vi "Prober_LoadUnload.vi"(8 "error in (no error)":errorcluster, 11 "TeslaVeloxProbeStation in":refnum<class "TeslaVeloxProbeStation.lvclass">) -> (0 "error out":errorcluster, 2 "Home or Load?":enum16{"Measure", "Load"}(ring), 3 "TeslaVeloxProbeStation out":refnum<class "TeslaVeloxProbeStation.lvclass">)   [LabVIEW 2018, in "TeslaVeloxProbeStation.lvclass"]
uses:
  TeslaVeloxProbeStation.lvclass
  Desktop/Kvasnicka/test_labview_library/Integration_toolkit_library/CascadeProbestation.lvlib
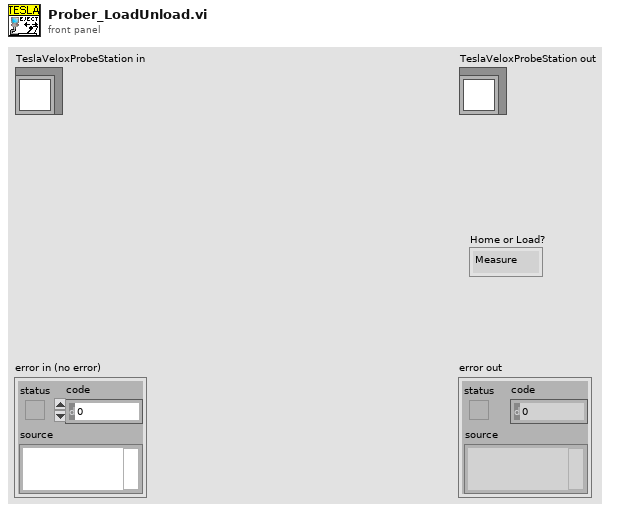
[diagram p1: front panel]
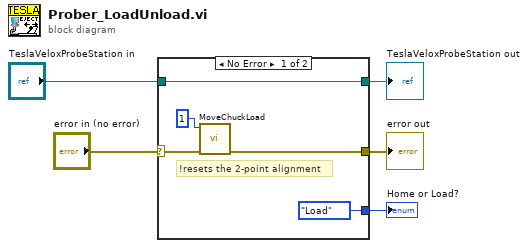
[diagram p0: block diagram]
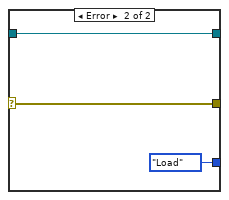
[diagram p2: hidden frame]
diagram:
  n1 = case shown="No Error" "error in (no error)" {
    selector: "error in (no error)" -> [w8 w12]
    tunnel: [enum16{"Measure", "Load"}."Load" ("Home or Load?") enum16{"Measure", "Load"}."Load" ("Home or Load?")] -> w4
    tunnel: [w7 w12] -> w3
    tunnel: [w6 w13] -> w2
    tunnel: "TeslaVeloxProbeStation in" -> [w6 w13]
    frame No Error {
      # "!resets the 2-point alignment"
      n2 = call "MoveChuckLoad.vi"("Error In"=w8, "Load position"=1) -> ("Error Out"=w7:errorcluster)  [unwired: 8 in, 1 out]
    }
    frame Error {
    }
  }
  "error out" <- w3
  "Home or Load?" <- w4
  "TeslaVeloxProbeStation out" <- w2
